vi "Fail if Match.vi"(8 "error in (no error)":errorcluster, 10 "regular expression":string, 11 "XML Report Test in":refnum<class "Text Report Test.lvclass">) -> (0 "error out":errorcluster, 1 "Report Content":string, 3 "XML Report Test out":refnum<class "Text Report Test.lvclass">)   [LabVIEW 2020, in "Text Report Test.lvclass"]
uses:
  Text Report Test.lvclass
  Text Report Test.lvclass/Text Report Test.ctl
  <vilib>/Astemes/LUnit/Test Case.lvclass
  C:/Program Files (x86)/National Instruments/LabVIEW 2020/vi.lib/Astemes/LUnit/Test Case.lvclass
  C:/git/astemes-lunit/tests/Text Report Test/Text Report Test.lvclass
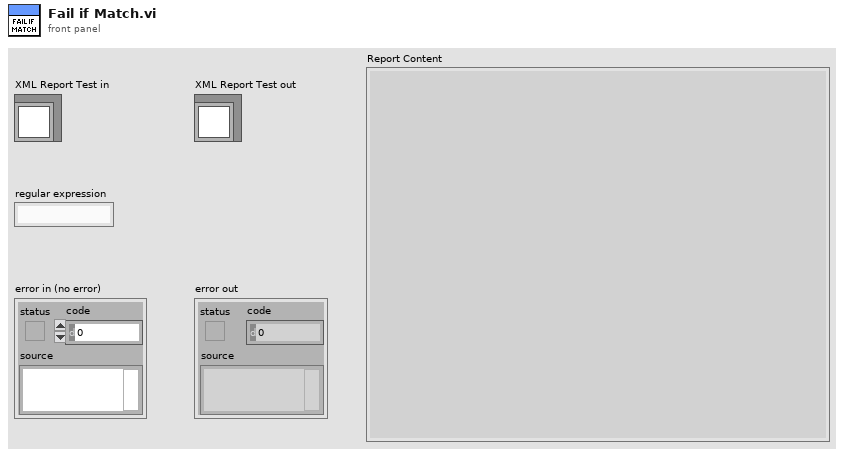
[diagram p1: front panel]
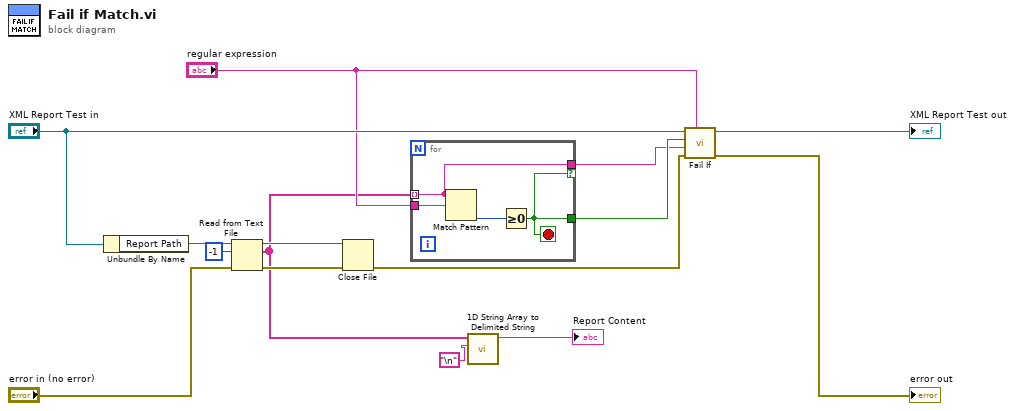
[diagram p0: block diagram]
diagram:
  n1 = Unbundle By Name("XML Report Test in") -> ("Report Path"=w12:path)
  n2 = Read from Text File(file (use dialog)=w12, count=-1, error in="error in (no error)") -> (refnum out=w10:refnum<file>, text=w4:string[], error out=w11:errorcluster)  [unwired: 1 in, 1 out]
  n3 = Close File(refnum=w10, error in=w11) -> (error out=w7:errorcluster)  [unwired: 1 out]
  n4 = for {
    tunnel: [w16] -> w9
    tunnel: "regular expression" -> [w18]
    tunnel: w4 -> [w17] mode=indexing
    tunnel: [w17] -> w3 if=w16
    stop <- w16 stop-if-true
    n5 = Match Pattern(string=w17, regular expression=w18) -> (offset past match=w19:i32)  [unwired: 1 in, 3 out]
    n6 = Greater Or Equal To 0?(x=w19) -> (x >= 0?=w16:bool)
  }
  n7 = call <vilib>:"1D String Array to Delimited String.vi"("delimiter"="\n", "string array"=w4) -> ("delimited string"=→"Report Content":string)  [unwired: 9 in]
  n8 = call <vilib>:"Fail If.vi"("Description"="regular expression", "error in (no error)"=w7, "Message"=w3, "Fail?"=w9, "LUnit Test Case In"="XML Report Test in") -> ("error out"=→"error out":errorcluster, "LUnit Test Case Out"=→"XML Report Test out":refnum<class "Text Report Test.lvclass">)  [unwired: 5 in]
